vi "Day 9 - Mirage Maintenance.vi"() -> ()   [LabVIEW 2020, in "AoC 2023.lvlib"]
uses:
  AoC 2023.lvlib
panel:
  out "Puzzle Part-2 Answer":string
  out "Puzzle Answer":string
  in  "Puzzle Input":string="0 3 6 9 12 15\n1 3 6 10 15 21\n10 13 16 21 30 45"
  # "Enter the Puzzle Input and run the VI"
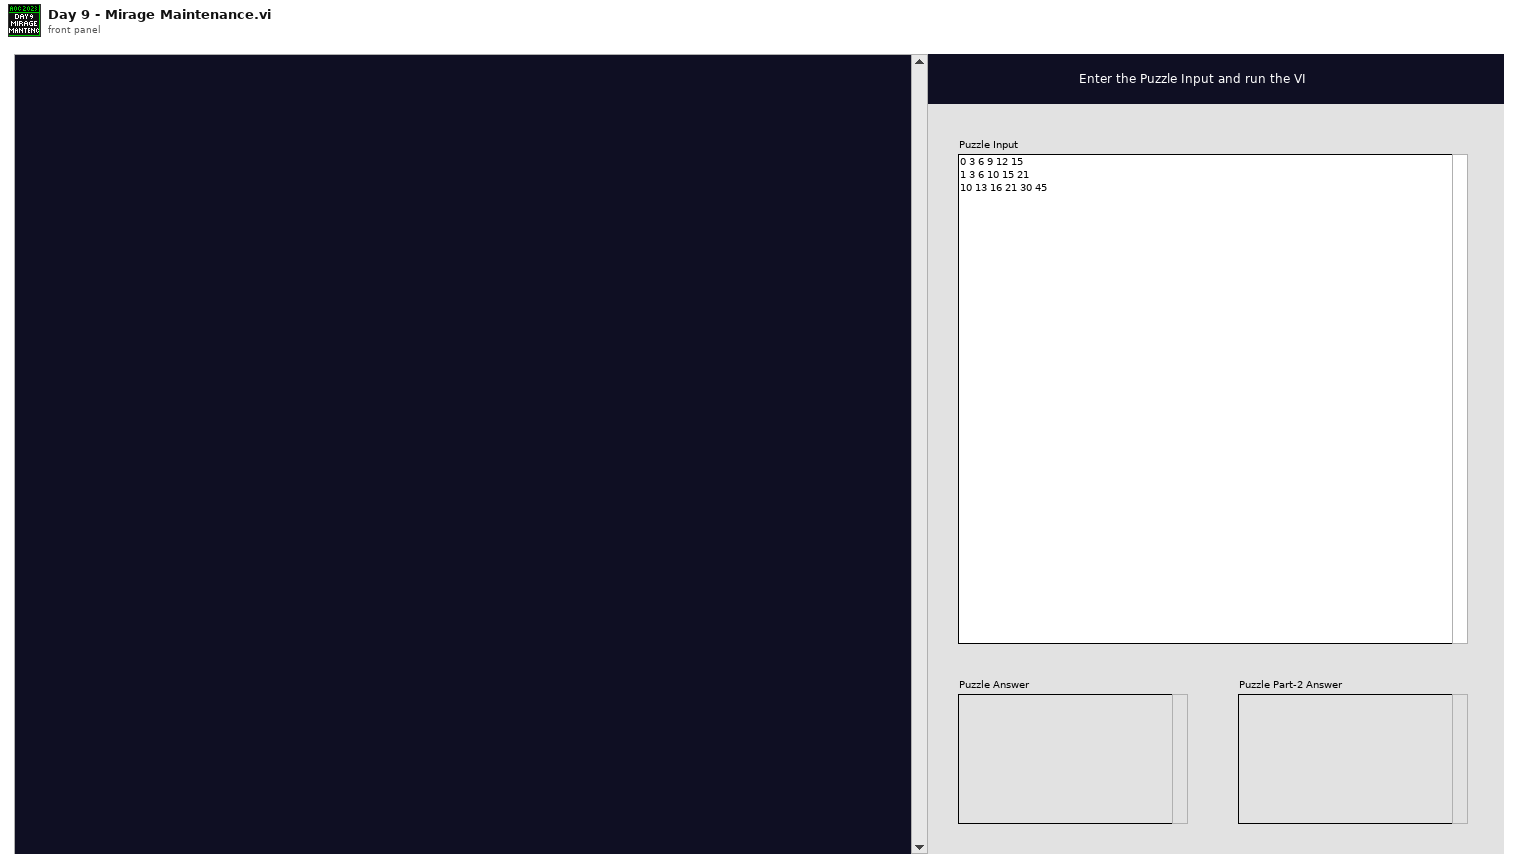
[diagram p1: front panel]
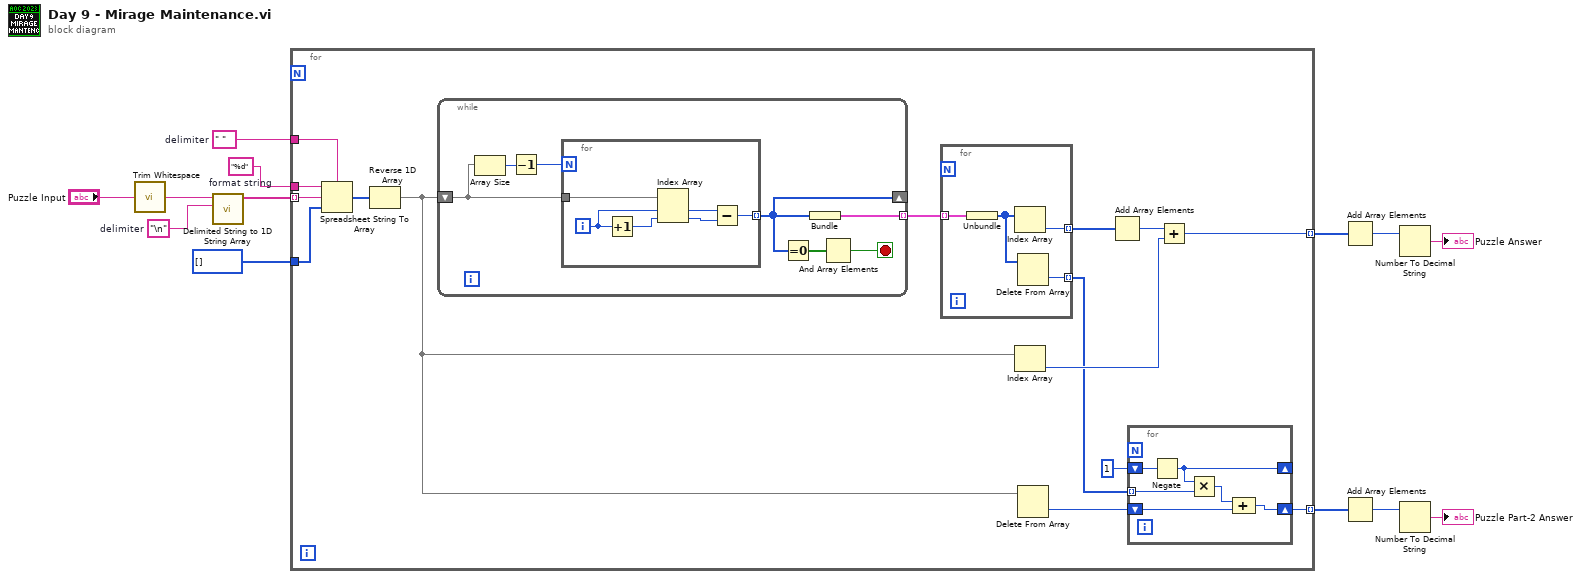
[diagram p0: block diagram]
diagram:
  w2 = "%d"  # format string
  w4 = " "  # delimiter
  w10 = "\n"  # delimiter
  n1 = call <vilib>:"Trim Whitespace.vi"("string"="Puzzle Input") -> ("trimmed string"=w9:string)  [unwired: 1 in]
  n2 = call <vilib>:"Delimited String to 1D String Array.vi"("delimiter"=w10, "delimited string"=w9) -> ("string array"=w1:string[])  [unwired: 9 in]
  n3 = for {
    tunnel: [w25] -> w8 mode=indexing
    tunnel: [w20] -> w5 mode=indexing
    tunnel: w4 -> [w18]
    tunnel: i64[] [] -> [w17]
    tunnel: w2 -> [w16]
    tunnel: w1 -> [w15] mode=indexing
    n4 = Spreadsheet String To Array(delimiter (Tab)=w18, format string=w16, spreadsheet string=w15, array type (2D Dbl)=w17) -> (array=w19:i64[])
    n5 = Reverse 1D Array(array=w19) -> (reversed array=w14:i64[])
    n6 = while {
      tunnel: [w41] -> w24 mode=indexing
      shift-right: [w39] -> _
      shift-left: w14 -> [w43]
      stop <- w40 stop-if-true
      n7 = Array Size(array=w43) -> (size(s)=w45:i32)
      n8 = Decrement(x=w45) -> (x-1=w44:i32)
      n9 = for {
        N: w44 -> [_]
        tunnel: w43 -> [w51]
        tunnel: [w46] -> w39 mode=indexing
        i -> [w50]
        n10 = Increment(x=w50) -> (x+1=w49:i32)
        n11 = Index Array(array=w51, index #1=w50, index #2=w49) -> (element #1=w48:i64, element #2=w47:i64)
        n12 = Subtract(x=w48, y=w47) -> (x-y=w46:i64)
      }
      n13 = Equal To 0?(x=w39) -> (x = 0?=w42:bool[])
      n14 = Bundle(w39) -> (w41:cluster{i64[]})  [unwired: 1 in]
      n15 = And Array Elements(Boolean array=w42) -> (logical AND=w40:bool)
    }
    n16 = for {
      tunnel: w24 -> [w38] mode=indexing
      tunnel: [w37] -> w28 mode=indexing
      tunnel: [w35] -> w23 mode=indexing
      n17 = Unbundle(w38) -> (w36:i64[])
      n18 = Index Array(array=w36) -> (element=w37:i64)  [unwired: 1 in]
      n19 = Delete From Array(array=w36) -> (deleted portion=w35:i64)  [unwired: 2 in, 1 out]
    }
    n20 = Index Array(array=w14) -> (element=w26:i64)  [unwired: 1 in]
    n21 = Delete From Array(array=w14) -> (deleted portion=w22:i64)  [unwired: 2 in, 1 out]
    n22 = Add Array Elements(numeric array=w28) -> (sum=w27:i64)
    n23 = for {
      tunnel: w23 -> [w32] mode=indexing
      shift-right: [w33] -> w20
      shift-left: w22 -> [w34]
      shift-right: [w30] -> _
      shift-left: i64 1 -> [w29]
      n24 = Negate(x=w29) -> (-x=w30:i64)
      n25 = Multiply(x=w30, y=w32) -> (x*y=w31:i64)
      n26 = Compound Arithmetic op=ADD(w31, w34) -> (w33:i64)
    }
    n27 = Add(x=w27, y=w26) -> (x+y=w25:i64)
  }
  n28 = Add Array Elements(numeric array=w8) -> (sum=w7:i64)
  n29 = Add Array Elements(numeric array=w5) -> (sum=w6:i64)
  n30 = Number To Decimal String(number=w7) -> (decimal integer string=→"Puzzle Answer":string)  [unwired: 1 in]
  n31 = Number To Decimal String(number=w6) -> (decimal integer string=→"Puzzle Part-2 Answer":string)  [unwired: 1 in]
